vi "Operator Panel 2D_final.vi"() -> ()   [LabVIEW 2016]
doc: "This VI is an example operator panel.\n\nThe VI contains a table for the field values that may be configured manually, or loaded by checking the \"Prompt for File\" box. The data file should contain 3 columns of data, with each column delimited by a tab character.\n\nBefore the VI is executed, set the desired field units and coordinate system. Once the VI is started, follow the directions in the STATUS indicator to operate. Once a field value is achieved, it will be held indefinitely with no user intervention.\n\nThe present field is displayed in the selected units and coordinate system. The present field is queried once per second.\n\nIf a field point is specified that is outside the limits for the magnet, the VI will abort execution."
uses:
  <vilib>/Utility/file.llb/Read From Spreadsheet File (DBL).vi
panel:
  out "Number of lines":i32=5
  in  "Starting index 2":i32=8 min=0 max=17 step=1
  in  "Operation":u16(ring)=1 items=["Stepwise", "Continous"]
  out "Ramp Rate along Vector (T/min)":dbl=0.17756501513530193 format="%.3f"
  out "Current Ramp Rate Z (T/min)":dbl=0.00639 format="%.3f"
  out "Current Ramp Rate Y (T/min)":dbl=0.17745 format="%.3f"
  in  "User defined Ramp Rate (T/min)":bool
  in  "User defined Ramp Rate (T/min)":dbl=0.178 format="%.3f"
  in  "Z-Axis Communications Config":T1={"GPIB address"=22, "GPIB bus"=1, "connection ID"=refnum, "IP"="111.111.111.1", "Active Comm Interface"=0, "Serial Port"="", "Programmer Type"=0} {"Programmer Type" items=["Model 430", "Model 420"]; "Active Comm Interface" items=["TCP/IP (Model 430 Only)", "RS232", "IEEE488"]}
  in  "Max Ramp Rate - Y Axis (A/s)":dbl=0.065 format="%.3f"
  in  "Max Ramp Rate - Z Axis (A/s)":dbl=0.203 format="%.3f"
  in  "Magnitude Limit (kG)":dbl=45.1 format="%.3f"
  in  "Y-Axis Communications Config":T1={"GPIB address"=22, "GPIB bus"=1, "connection ID"=refnum, "IP"="111.111.111.2", "Active Comm Interface"=0, "Serial Port"="", "Programmer Type"=0} {"Programmer Type" items=["Model 430", "Model 420"]; "Active Comm Interface" items=["TCP/IP (Model 430 Only)", "RS232", "IEEE488"]}
  out "Cartesian Display (T)":T2={"Y-Axis Field (T)"=-1e-05, "Z-Axis Field (T)"=-0.0} {"Z-Axis Field (T)" format="%.3f"; "Y-Axis Field (T)" format="%.3f"}
  in  "Starting index":i32=5
  in  "Normal color":u32(colorbox)=11711154
  in  "Highlight color":u32(colorbox)=16711680
  out "?":string="American Magnetics, Inc."
  in  "Prompt for File?":bool
  out "Continue Execution?":bool=TRUE
  out "error out":T3
  in  "error in":T3
  out "STATUS":string="Holding at current vector. Set Ramping Mode to NEXT VECTOR to continue."
  in  "Ramping Control":u16(ring)=2 items=["NEXT VECTOR", "RAMPING", "HOLDING", "PAUSE", "ZERO"]
  out "Cartesian Display (kG)":T4 {"Z-Axis Field (kG)" format="%.3f"; "Y-Axis Field (kG)" format="%.3f"}
  in  "Field Values":string[][](table)=[["0", "0"], ["0", "-9"], ["0", "0"], ["4.5", "0"], ["0", "0"]]
  out "Switch Heaters":bool=TRUE
  out "Polar Display (T)":T5={"q (degrees)"=340.4633450618716, "Field Magnitude (T)"=0.09999705595666304} {"Field Magnitude (T)" format="%.3f"; "q (degrees)" format="%.3f"}
  out "Polar Display (kG)":T6 {"Field Magnitude (kG)" format="%.3f"; "q (degrees)" format="%.3f"}
  in  "Coordinate System":u16(ring) items=["Cartesian", "Polar"]
  in  "Magnetic Field Units":u16(ring)=1 items=["kG", "Tesla"]
  # "Configuration and Status"
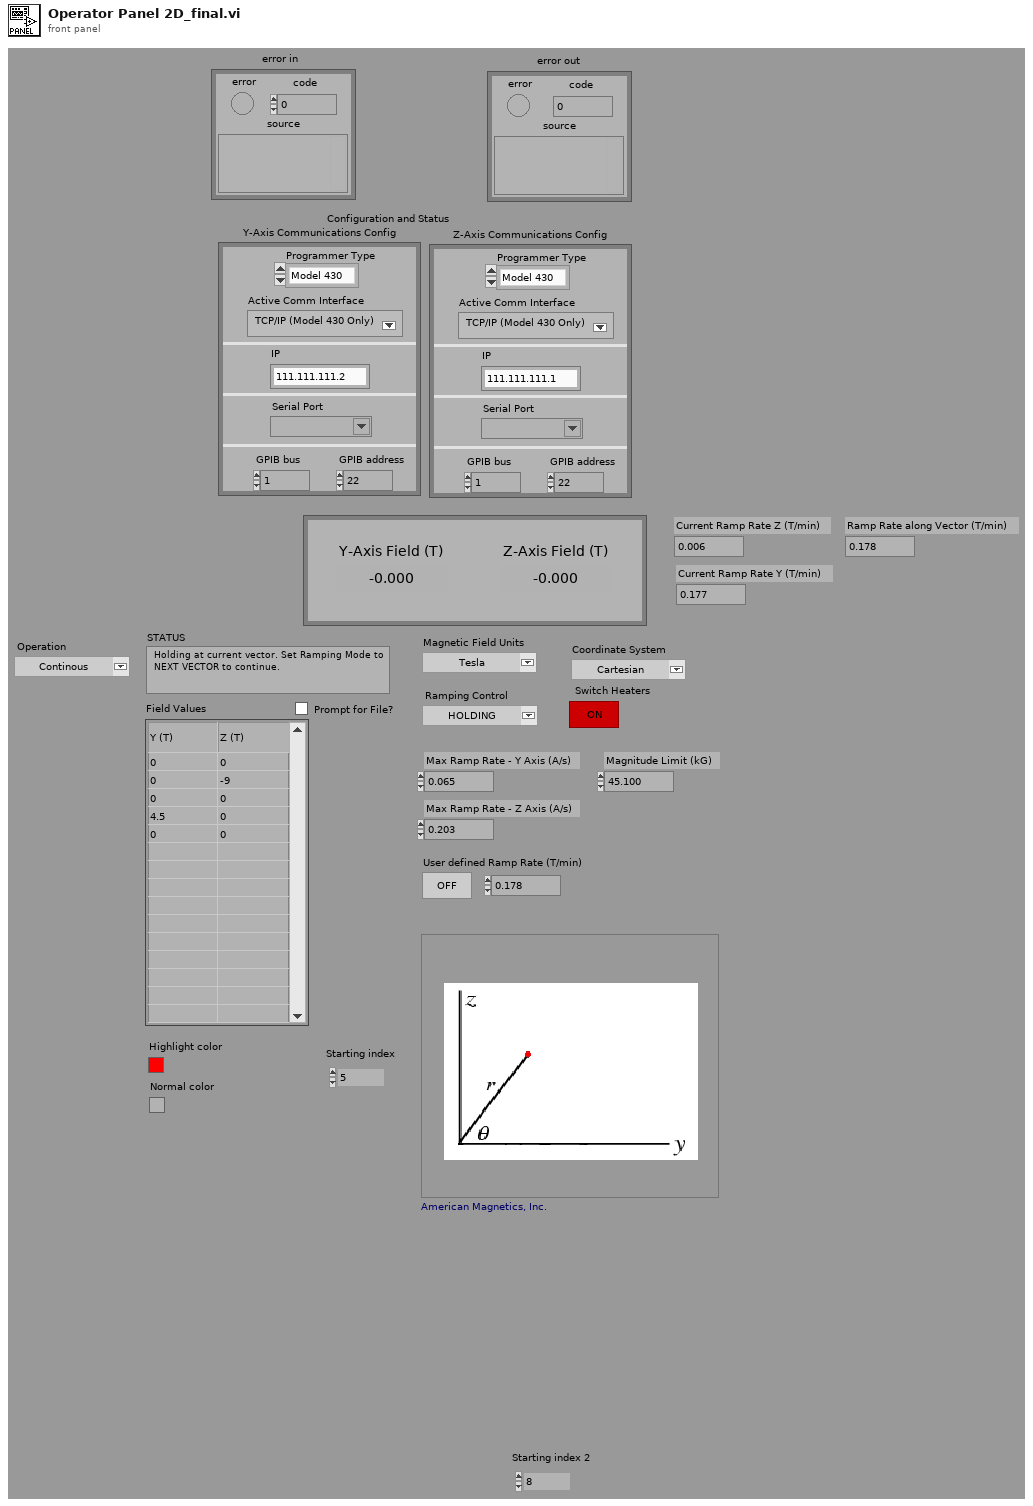
[diagram p1: front panel]
types:
  T1 = cluster{"GPIB address":i16, "GPIB bus":i16, "connection ID":refnum<k5>, "IP":string, "Active Comm Interface":u16, "Serial Port":refnum<visa-resource-name>, "Programmer Type":u16}
  T2 = cluster{"Y-Axis Field (T)":dbl, "Z-Axis Field (T)":dbl}
  T3 = cluster{"error":bool, "code":i32, "source":string}
  T4 = cluster{"Y-Axis Field (kG)":dbl, "Z-Axis Field (kG)":dbl}
  T5 = cluster{"q (degrees)":dbl, "Field Magnitude (T)":dbl}
  T6 = cluster{"q (degrees)":dbl, "Field Magnitude (kG)":dbl}
  T7 = enum16{"", "RAMPING", "HOLDING", "PAUSED", "MANUAL UP", "MANUAL DOWN", "ZEROING CURRENT", "QUENCH DETECTED", "HEATING SWITCH"}
  T8 = enum16{"", "RAMPING", "HOLDING", "PAUSED", "MANUAL UP", "MANUAL DOWN", "ZEROING CURRENT", "QUENCH DETECTED", "HEATING SWITCH", "AT ZER0", "COOLING SWITCH"}
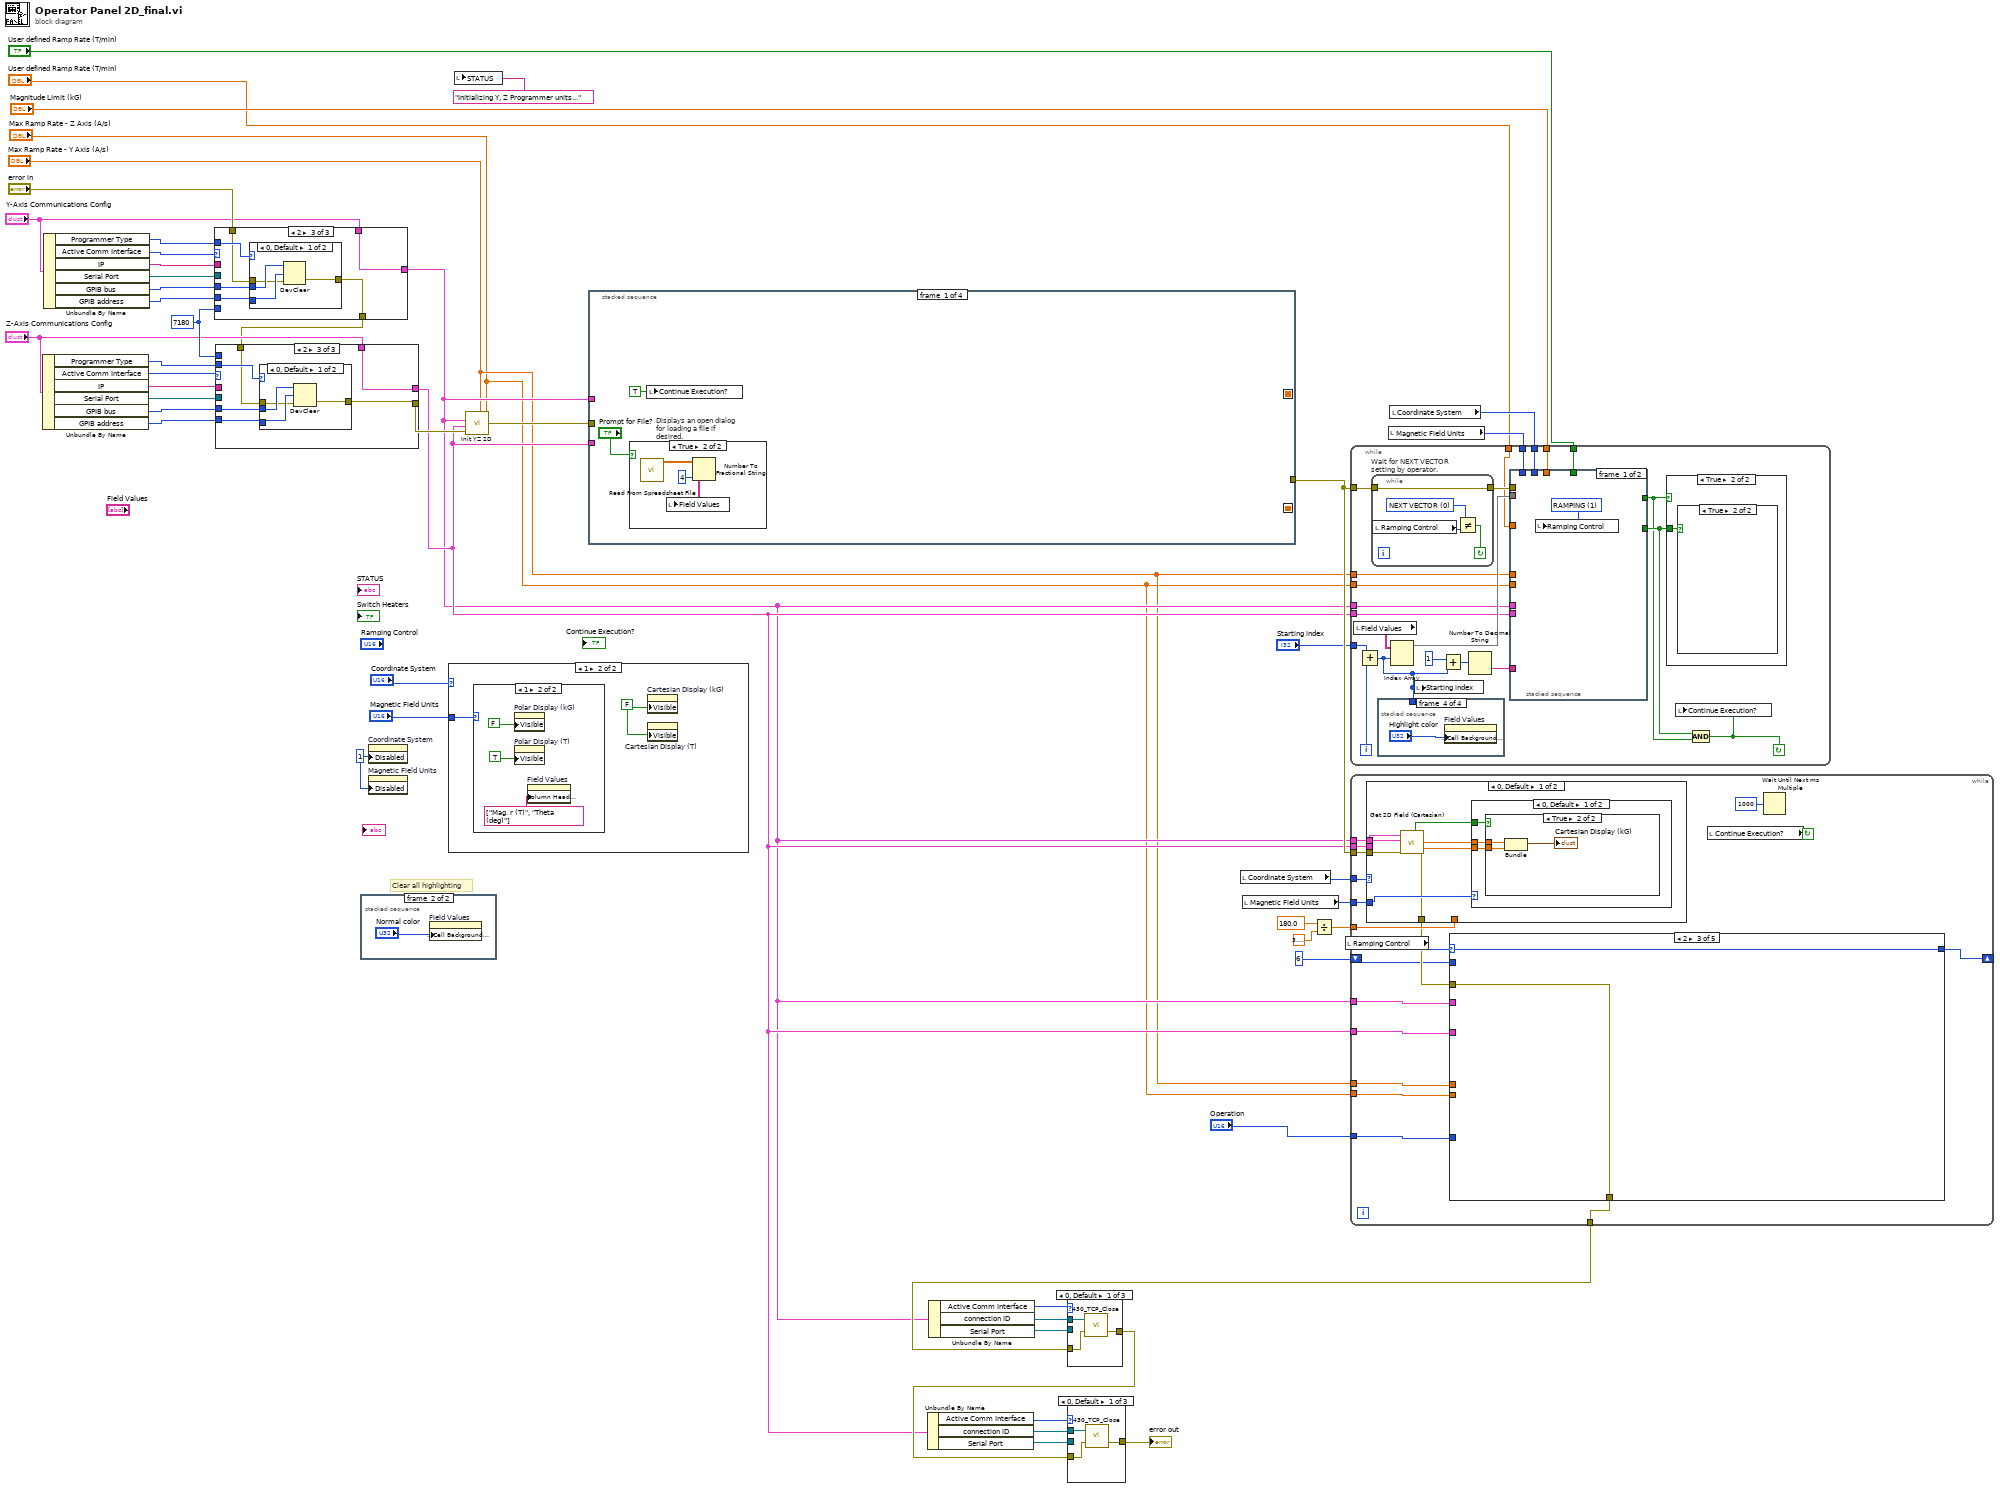
[diagram p0: block diagram]
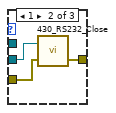
[diagram p2: hidden frame]
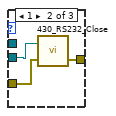
[diagram p4: hidden frame]
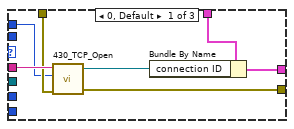
[diagram p6: hidden frame]
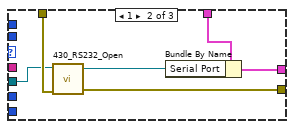
[diagram p7: hidden frame]
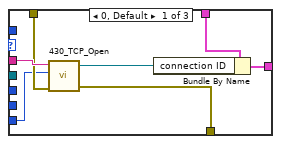
[diagram p9: hidden frame]
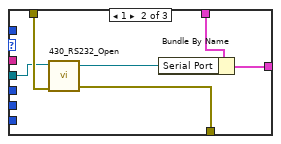
[diagram p10: hidden frame]
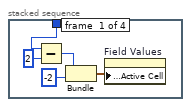
[diagram p12: hidden frame]
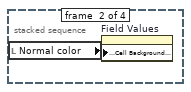
[diagram p13: hidden frame]
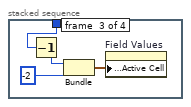
[diagram p14: hidden frame]
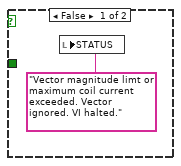
[diagram p15: hidden frame]
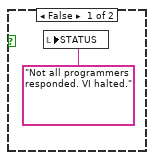
[diagram p16: hidden frame]
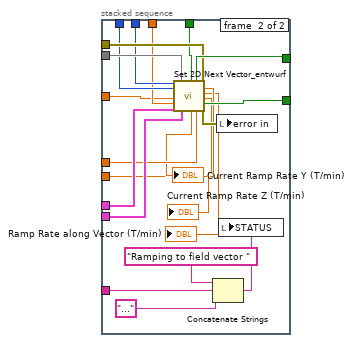
[diagram p17: hidden frame]
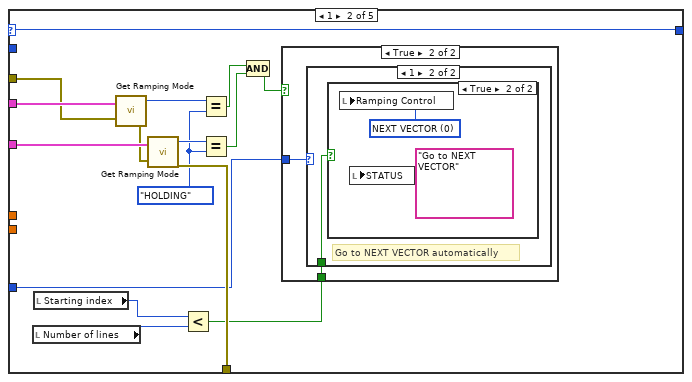
[diagram p19: hidden frame]
diagram:
  w35 = 7180 ("TCP Port")
  w48 = u8 1 ("Write Attribute")
  # "Clear all highlighting"
  n1 = Unbundle By Name("Z-Axis Communications Config") -> ("Programmer Type"=w10:u16, "Active Comm Interface"=w34:u16, "IP"=w31:string, "Serial Port"=w30:refnum<visa-resource-name>, "GPIB bus"=w9:i16, "GPIB address"=w8:i16)
  n2 = Unbundle By Name("Y-Axis Communications Config") -> ("Programmer Type"=w4:u16, "Active Comm Interface"=w33:u16, "IP"=w32:string, "Serial Port"=w29:refnum<visa-resource-name>, "GPIB bus"=w5:i16, "GPIB address"=w6:i16)
  n3 = case shown="2" w33 {
    tunnel: w32 -> [w57 _ _]
    tunnel: "error in" -> [w56 w63 w65]
    tunnel: "Y-Axis Communications Config" -> [w55 w58 w69]
    tunnel: [w53 w61 w69] -> w17
    tunnel: [w52 w62 w64] -> w7
    tunnel: w35 -> [w51 _ _]
    tunnel: w29 -> [_ w59 _]
    tunnel: w6 -> [_ _ w68]
    tunnel: w5 -> [_ _ w67]
    tunnel: w4 -> [_ _ w66]
    frame 0, Default {
      n4 = call "430_TCP_Open.vi"("IP Address"=w57, "TCP Port"=w51, "error in (no error)"=w56) -> ("connection ID"=w54:refnum<k5>, "error out"=w52:errorcluster)  [unwired: 3 in, 1 out]
      n5 = Bundle By Name(cluster=w55, "connection ID"=w54) -> (w53:T1)
    }
    frame 1 {
      n6 = call "430_RS232_Open.vi"("VISA resource name"=w59, "error in (no error)"=w63) -> ("VISA resource name out"=w60:refnum<visa-resource-name>, "error out"=w62:errorcluster)  [unwired: 5 in]
      n7 = Bundle By Name(cluster=w58, "Serial Port"=w60) -> (w61:T1)
    }
    frame 2 {
      n8 = case shown="0, Default" w66 {
        tunnel: w67 -> [w73 _]
        tunnel: w68 -> [w72 _]
        tunnel: w65 -> [w71 w74]
        tunnel: [w70 w74] -> w64
        frame 0, Default {
          n9 = DevClear(2:w71, 3:w72, 4:w73) -> (0:w70:errorcluster)  [unwired: 1 out]
        }
        frame 1 {
        }
      }
    }
  }
  n10 = case shown="2" w34 {
    tunnel: w31 -> [w81 _ _]
    tunnel: w7 -> [w80 w87 w89]
    tunnel: [w79 w86 w88] -> w27
    tunnel: "Z-Axis Communications Config" -> [w78 w84 w93]
    tunnel: [w76 w85 w93] -> w18
    tunnel: w35 -> [w75 _ _]
    tunnel: w30 -> [_ w82 _]
    tunnel: w10 -> [_ _ w92]
    tunnel: w9 -> [_ _ w91]
    tunnel: w8 -> [_ _ w90]
    frame 0, Default {
      n11 = call "430_TCP_Open.vi"("IP Address"=w81, "TCP Port"=w75, "error in (no error)"=w80) -> ("connection ID"=w77:refnum<k5>, "error out"=w79:errorcluster)  [unwired: 3 in, 1 out]
      n12 = Bundle By Name(cluster=w78, "connection ID"=w77) -> (w76:T1)
    }
    frame 1 {
      n13 = call "430_RS232_Open.vi"("VISA resource name"=w82, "error in (no error)"=w87) -> ("VISA resource name out"=w83:refnum<visa-resource-name>, "error out"=w86:errorcluster)  [unwired: 5 in]
      n14 = Bundle By Name(cluster=w84, "Serial Port"=w83) -> (w85:T1)
    }
    frame 2 {
      n15 = case shown="0, Default" w92 {
        tunnel: w91 -> [w97 _]
        tunnel: w90 -> [w96 _]
        tunnel: w89 -> [w95 w98]
        tunnel: [w94 w98] -> w88
        frame 0, Default {
          n16 = DevClear(2:w95, 3:w96, 4:w97) -> (0:w94:errorcluster)  [unwired: 1 out]
        }
        frame 1 {
        }
      }
    }
  }
  n17 = stacked-sequence {
    frame #0 {
      w99 = -2
      n18 = Bundle(w99, w99) -> (w100:cluster{i32, i32})  [unwired: 1 in]
      n19 = property on="Field Values" class="Tbl (strict)"("Active Cell:Active Cell"=w100) -> ()  [unwired: 2 in, 2 out]
    }
    frame #1 {
      n20 = property on="Field Values" class="Tbl (strict)"("Active Cell:Cell Background Color"="Normal color") -> ()  [unwired: 2 in, 2 out]
    }
  }
  n21 = property on="Coordinate System" class="Ring (strict)"("Disabled"=w48) -> ()  [unwired: 2 in, 2 out]
  n22 = property on="Magnetic Field Units" class="Ring (strict)"("Disabled"=w48) -> ()  [unwired: 2 in, 2 out]
  n23 = case shown="1" "Coordinate System" {
    tunnel: "Magnetic Field Units" -> [w103 w111]
    frame 0, Default {
      w102 = FALSE ("Write Attribute")
      (unwired) FALSE ("Write Attribute")
      (unwired) TRUE ("Write Attribute")
      n24 = case shown="0, Default" w103 {
        frame 0, Default {
          n25 = property on="Cartesian Display (kG)" class="Clust (strict)"("Visible"=TRUE ("Write Attribute")) -> ()  [unwired: 2 in, 2 out]
          n26 = property on="Cartesian Display (T)" class="Clust (strict)"("Visible"=FALSE ("Write Attribute")) -> ()  [unwired: 2 in, 2 out]
          n27 = property on="Field Values" class="Tbl (strict)"("Column Header Strings[]"=string[] ["Y (KG)", "Z (KG)"] ("Write Attribute")) -> ()  [unwired: 2 in, 2 out]
        }
        frame 1 {
          n28 = property on="Cartesian Display (kG)" class="Clust (strict)"("Visible"=FALSE ("Write Attribute")) -> ()  [unwired: 2 in, 2 out]
          n29 = property on="Cartesian Display (T)" class="Clust (strict)"("Visible"=TRUE ("Write Attribute")) -> ()  [unwired: 2 in, 2 out]
          n30 = property on="Field Values" class="Tbl (strict)"("Column Header Strings[]"=string[] ["Y (T)", "Z (T)"] ("Write Attribute")) -> ()  [unwired: 2 in, 2 out]
        }
      }
      n31 = property on="Polar Display (kG)" class="Clust (strict)"("Visible"=w102) -> ()  [unwired: 2 in, 2 out]
      n32 = property on="Polar Display (T)" class="Clust (strict)"("Visible"=w102) -> ()  [unwired: 2 in, 2 out]
    }
    frame 1 {
      (unwired) FALSE ("Write Attribute")
      (unwired) TRUE ("Write Attribute")
      w110 = FALSE ("Write Attribute")
      n33 = case shown="1" w111 {
        frame 0, Default {
          n34 = property on="Polar Display (kG)" class="Clust (strict)"("Visible"=TRUE ("Write Attribute")) -> ()  [unwired: 2 in, 2 out]
          n35 = property on="Polar Display (T)" class="Clust (strict)"("Visible"=FALSE ("Write Attribute")) -> ()  [unwired: 2 in, 2 out]
          n36 = property on="Field Values" class="Tbl (strict)"("Column Header Strings[]"=string[] ["Mag. r (KG)", "Theta (deg)"] ("Write Attribute")) -> ()  [unwired: 2 in, 2 out]
        }
        frame 1 {
          n37 = property on="Polar Display (kG)" class="Clust (strict)"("Visible"=FALSE ("Write Attribute")) -> ()  [unwired: 2 in, 2 out]
          n38 = property on="Polar Display (T)" class="Clust (strict)"("Visible"=TRUE ("Write Attribute")) -> ()  [unwired: 2 in, 2 out]
          n39 = property on="Field Values" class="Tbl (strict)"("Column Header Strings[]"=string[] ["Mag. r (T)", "Theta (deg)"] ("Write Attribute")) -> ()  [unwired: 2 in, 2 out]
        }
      }
      n40 = property on="Cartesian Display (kG)" class="Clust (strict)"("Visible"=w110) -> ()  [unwired: 2 in, 2 out]
      n41 = property on="Cartesian Display (T)" class="Clust (strict)"("Visible"=w110) -> ()  [unwired: 2 in, 2 out]
    }
  }
  n42 = local write "STATUS"("Initializing Y, Z Programmer units..." ("STATUS")) -> ()
  n43 = call "Init YZ 2D.vi"("Max Ramp Rate Z-axis"="Max Ramp Rate - Z Axis (A/s)", "Max Ramp Rate Y-axis"="Max Ramp Rate - Y Axis (A/s)", "error in"=w27, "Z-Axis Communications Config"=w18, "Y-Axis Communications Config"=w17) -> ("error out"=w46:T3)  [unwired: 5 in]
  n44 = stacked-sequence {
    seq-local: [_ w125 _ _] -> [_ _ w172 _]
    seq-local: [_ w124 _ _] -> [_ _ w171 _]
    tunnel: w18 -> [_ w127 _ _]
    tunnel: w46 -> [_ w128 _ _]
    tunnel: [_ w123 _ _] -> w42
    tunnel: w17 -> [_ w126 _ _]
    frame #0 {
      n45 = case "Displays an open dialog for loading a file if desired." shown="True" "Prompt for File?" {
        frame False {
        }
        frame True {
          n46 = call-poly <vilib>:"Read From Spreadsheet File.vi"() -> ("all rows"=w122:dbl[][])  [unwired: 7 in, 4 out]
          n47 = Number To Fractional String(number=w122, precision (6)=i16 4) -> (F-format string=w121:string[][])  [unwired: 2 in]
          n48 = local write "Field Values"(w121) -> ()
        }
      }
      n49 = local write "Continue Execution?"(TRUE ("Continue Execution?")) -> ()
    }
    frame #1 {
      w136 = u16 3 items=["NEXT VECTOR", "RAMPING", "HOLDING", "PAUSE", "ZERO"] ("Ramping Control")
      n50 = call "Get Switch Present.vi"("error in"=w128, "Communications Config"=w126) -> ("error out"=w132:T3, "Switch Present?"=w133:bool)
      n51 = case shown="True" w133 {
        tunnel: w132 -> [w154 w163]
        tunnel: w126 -> [_ w156]
        tunnel: [0.0 w160] -> w124
        tunnel: [w154 w162] -> w131
        frame False {
        }
        frame True {
          n52 = call "Get Switch Heater Time.vi"("error in"=w163, "Communications Config"=w156) -> ("error out"=w159:T3, "Switch Heating Time (secs)"=w161:dbl)
          n53 = call "Get Switch Heater.vi"("error in"=w159, "Communications Config"=w156) -> ("error out"=w158:T3, "Switch Heater Indicator"=w157:bool)
          n54 = case shown="False" w157 {
            tunnel: [w168 w169] -> w162
            tunnel: w161 -> [w166 _]
            tunnel: [w166 0.0] -> w160
            tunnel: w158 -> [w164 w169]
            tunnel: w156 -> [w165 _]
            frame False {
              n55 = call "Set Switch Heater.vi"("error in"=w164, "Switch Heater Control"=TRUE, "Communications Config"=w165) -> ("error out"=w168:T3)
            }
            frame True {
            }
          }
        }
      }
      n56 = call "Get Switch Present.vi"("error in"=w131, "Communications Config"=w127) -> ("error out"=w129:T3, "Switch Present?"=w130:bool)
      n57 = case shown="True" w130 {
        tunnel: w129 -> [w137 w146]
        tunnel: w127 -> [_ w139]
        tunnel: [0.0 w143] -> w125
        tunnel: [w137 w145] -> w123
        frame False {
        }
        frame True {
          n58 = call "Get Switch Heater Time.vi"("error in"=w146, "Communications Config"=w139) -> ("error out"=w142:T3, "Switch Heating Time (secs)"=w144:dbl)
          n59 = call "Get Switch Heater.vi"("error in"=w142, "Communications Config"=w139) -> ("error out"=w141:T3, "Switch Heater Indicator"=w140:bool)
          n60 = case shown="False" w140 {
            tunnel: [w147 w152] -> w145
            tunnel: w144 -> [w150 _]
            tunnel: [w150 0.0] -> w143
            tunnel: w141 -> [w148 w152]
            tunnel: w139 -> [w149 _]
            frame False {
              n61 = call "Set Switch Heater.vi"("error in"=w148, "Switch Heater Control"=TRUE, "Communications Config"=w149) -> ("error out"=w147:T3)
            }
            frame True {
            }
          }
        }
      }
      n62 = local write "Ramping Control"(w136) -> ()
      n63 = local write "Switch Heaters"(TRUE ("Switch Heater Control")) -> ()
      n64 = property on="Switch Heaters" class="Bool (strict)"("Disabled"=u8 1 ("Write Attribute")) -> ()  [unwired: 2 in, 2 out]
    }
    frame #2 {
      n65 = Max & Min(x=w172, y=w171) -> (max(x,y)=w173:dbl)  [unwired: 1 out]
      n66 = local write "STATUS"("Heating switches..." ("STATUS")) -> ()
      n67 = Add(x=w173, y=2) -> (x+y=w177:dbl)
      n68 = property on="Ramping Control" class="Ring (strict)"("Disabled"=u8 1 ("Write Attribute")) -> ()  [unwired: 2 in, 2 out]
      n69 = Multiply(x=w177, y=1000) -> (x*y=w176:dbl)
      n70 = Wait (ms)(milliseconds to wait=w176) -> ()  [unwired: 1 out]
    }
    frame #3 {
      n71 = local write "STATUS"("Ready to ramp to first vector. Set Ramping Mode to NEXT VECTOR to begin." ("STATUS")) -> ()
      n72 = property on="Ramping Control" class="Ring (strict)"("Disabled"=u8 0 ("Write Attribute")) -> ()  [unwired: 2 in, 2 out]
      n73 = local read "Field Values"() -> (w182:string[][])
      n74 = Array Size(array=w182) -> (size(s)=w181:i32[])
      n75 = Index Array(array=w181, index=0) -> (element=→"Number of lines":i32)
    }
  }
  n76 = Unbundle By Name(w18) -> ("Active Comm Interface"=w24:u16, "connection ID"=w23:refnum<k5>, "Serial Port"=w22:refnum<visa-resource-name>)
  n77 = Unbundle By Name(w17) -> ("Active Comm Interface"=w25:u16, "connection ID"=w21:refnum<k5>, "Serial Port"=w20:refnum<visa-resource-name>)
  n78 = local read "Coordinate System"() -> (w43:u16)
  n79 = local read "Magnetic Field Units"() -> (w41:u16)
  n80 = Divide(x=180.0, y=3.141592653589793) -> (x/y=w38:dbl)
  n81 = while {
    shift-left: u16 6 ("Ramping Control") -> [w189]
    shift-right: [w190] -> _
    tunnel: [w192] -> w19
    tunnel: w18 -> [w194]
    tunnel: w17 -> [w195]
    tunnel: w38 -> [w197]
    tunnel: w41 -> [w198]
    tunnel: w42 -> [w199]
    tunnel: w18 -> [w200]
    tunnel: w17 -> [w201]
    tunnel: w43 -> [w202]
    tunnel: "Max Ramp Rate - Y Axis (A/s)" -> [w188]
    tunnel: "Max Ramp Rate - Z Axis (A/s)" -> [w187]
    tunnel: "Operation" -> [w186]
    stop <- w191 continue-if-true
    n82 = local read "Ramping Control"() -> (w196:u16)
    n83 = case shown="0, Default" w202 {
      tunnel: w201 -> [w276 w300]
      tunnel: w200 -> [w275 w299]
      tunnel: w199 -> [w274 w298]
      tunnel: w198 -> [w273 w297]
      tunnel: w197 -> [_ w294]
      tunnel: [w269 w292] -> w193
      frame 0, Default {
        n84 = call "Get 2D Field (Cartesian).vi"("Z-Axis Communications Config"=w276, 2:w275, "error in"=w274) -> ("All Instruments Responded?"=w270:bool, "Y-Axis Field (kG)"=w272:dbl, "Z-Axis Field (kG)"=w271:dbl, "error out"=w269:T3)  [unwired: 2 in]
        n85 = case shown="0, Default" w273 {
          tunnel: w272 -> [w279 w285]
          tunnel: w271 -> [w278 w286]
          tunnel: w270 -> [w277 w288]
          frame 0, Default {
            n86 = case shown="True" w277 {
              tunnel: w279 -> [_ w281]
              tunnel: w278 -> [_ w280]
              frame False {
              }
              frame True {
                n87 = Bundle("Y-Axis Field (kG)"=w281, "Z-Axis Field (kG)"=w280) -> (→"Cartesian Display (kG)":T4)  [unwired: 1 in]
              }
            }
          }
          frame 1 {
            w287 = 0.1 ("y")
            n88 = Multiply(x=w285, y=w287) -> (x*y=w284:dbl)
            n89 = Multiply(x=w286, y=w287) -> (x*y=w283:dbl)
            n90 = case shown="True" w288 {
              tunnel: w284 -> [_ w291]
              tunnel: w283 -> [_ w290]
              frame False {
              }
              frame True {
                n91 = Bundle(w291, w290) -> (→"Cartesian Display (T)":cluster{dbl, dbl})  [unwired: 1 in]
              }
            }
          }
        }
      }
      frame 1 {
        n92 = call "Get 2D Field (Polar).vi"("Y-Axis Communications Config"=w300, "Z-Axis Communications Config"=w299, "error in"=w298) -> ("All Instruments Responded?"=w293:bool, "Radial (r) Field (kG)"=w296:dbl, "q (radians)"=w295:dbl, "error out"=w292:T3)  [unwired: 2 in]
        n93 = case shown="1" w297 {
          tunnel: w296 -> [w305 w314]
          tunnel: w295 -> [w303 w313]
          tunnel: w294 -> [w302 w312]
          tunnel: w293 -> [w304 w311]
          frame 0, Default {
            n94 = Multiply(x=w303, y=w302) -> (x*y=w301:dbl)
            n95 = case shown="True" w304 {
              tunnel: w305 -> [_ w306]
              tunnel: w301 -> [_ w307]
              frame False {
              }
              frame True {
                n96 = Bundle(w307, "Radial (r) Field (kG)"=w306) -> (→"Polar Display (kG)":cluster{dbl, "Radial (r) Field (kG)":dbl})  [unwired: 1 in]
              }
            }
          }
          frame 1 {
            n97 = Multiply(x=w314, y=0.1) -> (x*y=w310:dbl)
            n98 = Multiply(x=w313, y=w312) -> (x*y=w309:dbl)
            n99 = case shown="True" w311 {
              tunnel: w310 -> [_ w316]
              tunnel: w309 -> [_ w317]
              frame False {
              }
              frame True {
                n100 = Bundle(w317, w316) -> (→"Polar Display (T)":cluster{dbl, dbl})  [unwired: 1 in]
              }
            }
          }
        }
      }
    }
    n101 = case shown="2" w196 {
      selector: w196 -> [w204 w218 w232 w235 w250]
      tunnel: w195 -> [_ w221 _ w239 w256]
      tunnel: w194 -> [_ w220 _ w238 w255]
      tunnel: w193 -> [w205 w213 w231 w237 w254]
      tunnel: [w205 w219 w231 w236 w253] -> w192
      tunnel: [w204 w218 w232 w235 w250] -> w190
      tunnel: w189 -> [_ _ _ w234 w252]
      tunnel: w188 -> [_ _ _ _ w249]
      tunnel: w187 -> [_ _ _ _ w248]
      tunnel: w186 -> [_ w209 _ _ _]
      frame 0, Default {
      }
      frame 1 {
        w212 = T7."HOLDING" ("y")
        n102 = local read "Number of lines"() -> (w206:i32)
        n103 = local read "Starting index"() -> (w208:i32)
        n104 = call "Get Ramping Mode.vi"("Communications Config"=w221, "error in"=w213) -> ("Ramping Mode"=w216:T8, "error out"=w217:T3)  [unwired: 1 out]
        n105 = call "Get Ramping Mode.vi"("Communications Config"=w220, "error in"=w217) -> ("Ramping Mode"=w215:T8, "error out"=w219:T3)  [unwired: 1 out]
        n106 = Less?(x=w208, y=w206) -> (x < y?=w207:bool)
        n107 = Equal?(x=w216, y=w212) -> (x = y?=w211:bool)
        n108 = Equal?(x=w215, y=w212) -> (x = y?=w210:bool)
        n109 = Compound Arithmetic op=AND(w211, w210) -> (w214:bool)
        n110 = case shown="True" w214 {
          tunnel: w209 -> [_ w223]
          tunnel: w207 -> [_ w222]
          frame False {
          }
          frame True {
            n111 = case shown="1" w223 {
              tunnel: w222 -> [_ w226]
              frame 0, Default {
                w225 = u16 2 items=["NEXT VECTOR", "RAMPING", "HOLDING", "PAUSE", "ZERO"] ("Ramping Control")
                n112 = local write "STATUS"("Holding at current vector. Set Ramping Mode to NEXT VECTOR to continue." ("STATUS")) -> ()
                n113 = local write "Ramping Control"(w225) -> ()
              }
              frame 1 {
                # "Go to NEXT VECTOR automatically"
                n114 = case shown="True" w226 {
                  frame False {
                    w228 = u16 2 items=["NEXT VECTOR", "RAMPING", "HOLDING", "PAUSE", "ZERO"] ("Ramping Control")
                    n115 = local write "STATUS"("Holding at current vector. Set Ramping Mode to NEXT VECTOR to continue." ("STATUS")) -> ()
                    n116 = local write "Ramping Control"(w228) -> ()
                  }
                  frame True {
                    w230 = u16 0 items=["NEXT VECTOR", "RAMPING", "HOLDING", "PAUSE", "ZERO"] ("Ramping Control")
                    n117 = local write "Ramping Control"(w230) -> ()
                    n118 = local write "STATUS"("Go to NEXT VECTOR" ("STATUS")) -> ()
                  }
                }
              }
            }
          }
        }
      }
      frame 2 {
      }
      frame 3 {
        n119 = Not Equal?(x=w235, y=w234) -> (x != y?=w233:bool)
        n120 = case shown="True" w233 {
          tunnel: w239 -> [_ w247]
          tunnel: w238 -> [_ w246]
          tunnel: w237 -> [w240 w241]
          tunnel: [w240 w244] -> w236
          frame False {
          }
          frame True {
            w242 = u16 1 items=["RAMP", "PAUSE", "MANUAL UP", "MANUAL DOWN", "ZERO"] ("Ramping Mode")
            n121 = call "Set Ramping Mode.vi"("error in"=w241, "Ramping Mode"=w242, "Communications Config"=w247) -> ("error out"=w245:T3)
            n122 = call "Set Ramping Mode.vi"("error in"=w245, "Ramping Mode"=w242, "Communications Config"=w246) -> ("error out"=w244:T3)
            n123 = local write "STATUS"("All Programmers are PAUSED. Set Ramping Mode to NEXT VECTOR to continue." ("STATUS")) -> ()
          }
        }
      }
      frame 4 {
        n124 = Not Equal?(x=w250, y=w252) -> (x != y?=w251:bool)
        n125 = case shown="True" w251 {
          tunnel: w256 -> [_ w264]
          tunnel: w255 -> [_ w263]
          tunnel: w254 -> [w257 w266]
          tunnel: [w257 w259] -> w253
          tunnel: w249 -> [_ w262]
          tunnel: w248 -> [_ w261]
          frame False {
          }
          frame True {
            w258 = u16 4 items=["RAMP", "PAUSE", "MANUAL UP", "MANUAL DOWN", "ZERO"] ("Ramping Mode")
            n126 = local write "STATUS"("Zeroing vector." ("STATUS")) -> ()
            n127 = call "Set Ramping Mode.vi"("error in"=w266, "Ramping Mode"=w258, "Communications Config"=w264) -> ("error out"=w268:T3)
            n128 = call "Set Ramping Mode.vi"("error in"=w268, "Ramping Mode"=w258, "Communications Config"=w263) -> ("error out"=w260:T3)
            n129 = call "Set Current Ramp Rate.vi"("Communications Config"=w264, "Ramp Rate (A/sec)"=w262, "error in"=w260) -> ("error out"=w265:T3)  [unwired: 2 in]
            n130 = call "Set Current Ramp Rate.vi"("Communications Config"=w263, "Ramp Rate (A/sec)"=w261, "error in"=w265) -> ("error out"=w259:T3)  [unwired: 2 in]
          }
        }
      }
    }
    n131 = local read "Continue Execution?"() -> (w191:bool)
    n132 = Wait Until Next ms Multiple(millisecond multiple=u32 1000) -> ()  [unwired: 1 out]
  }
  n133 = case shown="0, Default" w25 {
    tunnel: w21 -> [w321 _ _]
    tunnel: w19 -> [w320 w324 w325]
    tunnel: [w319 w323 w325] -> w26
    tunnel: w20 -> [_ w322 _]
    frame 0, Default {
      n134 = call "430_TCP_Close.vi"("error in (no error)"=w320, "connection ID"=w321) -> ("error out"=w319:errorcluster)  [unwired: 1 out]
    }
    frame 1 {
      n135 = call "430_RS232_Close.vi"("error in (no error)"=w324, "VISA resource name"=w322) -> ("error out"=w323:errorcluster)  [unwired: 1 in]
    }
    frame 2 {
    }
  }
  n136 = case shown="0, Default" w24 {
    tunnel: w23 -> [w328 _ _]
    tunnel: w26 -> [w327 w331 w332]
    tunnel: [w326 w330 w332] -> w16
    tunnel: w22 -> [_ w329 _]
    frame 0, Default {
      n137 = call "430_TCP_Close.vi"("error in (no error)"=w327, "connection ID"=w328) -> ("error out"=w326:errorcluster)  [unwired: 1 out]
    }
    frame 1 {
      n138 = call "430_RS232_Close.vi"("error in (no error)"=w331, "VISA resource name"=w329) -> ("error out"=w330:errorcluster)  [unwired: 1 in]
    }
    frame 2 {
    }
  }
  "error out" <- w16
  n139 = local read "Magnetic Field Units"() -> (w44:u16)
  n140 = local read "Coordinate System"() -> (w45:u16)
  n141 = while {
    tunnel: "Starting index" -> [w340]
    tunnel: w18 -> [w346]
    tunnel: w17 -> [w347]
    tunnel: w44 -> [w348]
    tunnel: w45 -> [w349]
    tunnel: w42 -> [w352]
    tunnel: "Max Ramp Rate - Y Axis (A/s)" -> [w336]
    tunnel: "Max Ramp Rate - Z Axis (A/s)" -> [w335]
    tunnel: "Magnitude Limit (kG)" -> [w337]
    tunnel: "User defined Ramp Rate (T/min)" -> [w334]
    tunnel: "User defined Ramp Rate (T/min)" -> [w333]
    i -> [w339]
    stop <- w341 continue-if-true
    n142 = local read "Field Values"() -> (w343:string[][])
    n143 = Add(x=w340, y=w339) -> (x+y=w338:i32)
    n144 = while "Wait for NEXT VECTOR setting by operator." {
      tunnel: [w356] -> w351
      tunnel: w352 -> [w356]
      stop <- w357 continue-if-true
      w355 = u16 0 items=["NEXT VECTOR", "RAMPING", "HOLDING", "PAUSE", "ZERO"] ("Ramping Control")
      n145 = local read "Ramping Control"() -> (w358:u16)
      n146 = Not Equal?(x=w355, y=w358) -> (x != y?=w357:bool)
    }
    n147 = stacked-sequence {
      tunnel: w338 -> [w360 _ w366 _]
      frame #0 {
        (unwired) -2
        n148 = Subtract(x=w360, y=2) -> (x-y=w363:i32)
        n149 = Bundle(w363, -2) -> (w361:cluster{i32, i32})  [unwired: 1 in]
        n150 = property on="Field Values" class="Tbl (strict)"("Active Cell:Active Cell"=w361) -> ()  [unwired: 2 in, 2 out]
      }
      frame #1 {
        n151 = local read "Normal color"() -> (w364:u32)
        n152 = property on="Field Values" class="Tbl (strict)"("Active Cell:Cell Background Color"=w364) -> ()  [unwired: 2 in, 2 out]
      }
      frame #2 {
        n153 = Decrement(x=w366) -> (x-1=w365:i32)
        n154 = Bundle(w365, -2) -> (w368:cluster{i32, i32})  [unwired: 1 in]
        n155 = property on="Field Values" class="Tbl (strict)"("Active Cell:Active Cell"=w368) -> ()  [unwired: 2 in, 2 out]
      }
      frame #3 {
        n156 = property on="Field Values" class="Tbl (strict)"("Active Cell:Cell Background Color"="Highlight color") -> ()  [unwired: 2 in, 2 out]
      }
    }
    n157 = Index Array(array=w343, index (row)=w338) -> (element=w350:string[])  [unwired: 1 in]
    n158 = local write "Starting index"(w338) -> ()
    n159 = Add(x=1, y=w338) -> (x+y=w353:i32)
    n160 = Number To Decimal String(number=w353) -> (decimal integer string=w342:string)  [unwired: 1 in]
    n161 = stacked-sequence {
      tunnel: [_ w394] -> w344
      tunnel: [_ w393] -> w345
      tunnel: w351 -> [_ w389]
      tunnel: w350 -> [_ w388]
      tunnel: w349 -> [_ w387]
      tunnel: w348 -> [_ w386]
      tunnel: w347 -> [_ w385]
      tunnel: w346 -> [_ w384]
      tunnel: w342 -> [_ w383]
      tunnel: w337 -> [_ w381]
      tunnel: w336 -> [_ w380]
      tunnel: w335 -> [_ w375]
      tunnel: w334 -> [_ w379]
      tunnel: w333 -> [_ w378]
      frame #0 {
        w373 = u16 1 items=["NEXT VECTOR", "RAMPING", "HOLDING", "PAUSE", "ZERO"] ("Ramping Control")
        n162 = local write "Ramping Control"(w373) -> ()
      }
      frame #1 {
        n163 = call "Set 2D Next Vector_entwurf.vi"("Coordinate System"=w387, "Magnetic Field Units"=w386, 3:"User defined Ramp Rate (T/min)"=w378, "Magnitude Limit (kG)"=w381, "Y-Axis Communications Config"=w385, "Input Vector"=w388, "Z-Axis Communications Config"=w384, 10:"User defined Ramp Rate (T/min)"=w379, "Max Ramp Rate - Y Axis (A/s)"=w380, "error in"=w389, "Max Ramp Rate - Z Axis (A/s)"=w375) -> ("Y-Axis Ramp Rate (T/min)"=→"Current Ramp Rate Y (T/min)":dbl, "Within Limits?"=w394:bool, "Ramp Rate along Vector (T/min)"=→"Ramp Rate along Vector (T/min)":dbl, "Z-Axis Ramp Rate (T/min)"=→"Current Ramp Rate Z (T/min)":dbl, "All Instruments Responded?"=w393:bool, "error out"=w382:T3)  [unwired: 3 in]
        n164 = Concatenate Strings("Ramping to field vector " ("STATUS"), w383, "..." ("STATUS")) -> (w390:string)
        n165 = local write "error in"(w382) -> ()
        n166 = local write "STATUS"(w390) -> ()
      }
    }
    n167 = case shown="True" w344 {
      tunnel: w345 -> [_ w371]
      frame False {
        n168 = local write "STATUS"("Vector magnitude limt or maximum coil current exceeded. Vector ignored. VI halted." ("STATUS")) -> ()
      }
      frame True {
        n169 = case shown="True" w371 {
          frame False {
            n170 = local write "STATUS"("Not all programmers responded. VI halted." ("STATUS")) -> ()
          }
          frame True {
          }
        }
      }
    }
    n171 = Compound Arithmetic op=AND(w345, w344) -> (w341:bool)
    n172 = local write "Continue Execution?"(w341) -> ()
  }
